vi "STM Read Meta Data (UDP Ref).vi"(6 "Options":T4={"Ignore Timeout Error"=TRUE, "timeout ms (1000)"=1000, "max size (548)"=548}, 8 "error in":errorcluster, 11 "connection ID":refnum<k16>) -> (0 "error out":errorcluster, 1 "Meta data":T1[](array[typedef]), 3 "Connection Info Out":T2, 4 "data info":T3)   [LabVIEW 2010]
doc: "This VI reads the meta data information from a remote computer. Use this VI to retrieve the variable names and types that a remote computer exports.\n\nThis VI parses the data and returns a cluster containing the meta data information.\n\nCopyright 2015, 2016, 2017 National Instruments Corporation\n\nLicensed under the Apache License, Version 2.0 (the \"License\"); you may not use this file except in compliance with the License.\n\n You may obtain a copy of the License at\n\n http://www.apache.org/licenses/LICENSE-2.0\n\nUnless required by applicable law or agreed to in writing, software distributed under the License is distributed on an \"AS IS\" BASIS, WITHOUT WARRANTIES OR CONDITIONS OF ANY KIND, either express or implied.\n\nSee the License for the specific language governing permissions and limitations under the License."
uses:
  stm_UDP Read Options.ctl
  stm_UDP Data Info.ctl
  stm_UDP Connection Info.ctl
  stm_MetaDataElement.ctl
  UDP/Read Meta Data (UDP Clst).vi
  NI STM.lvlib
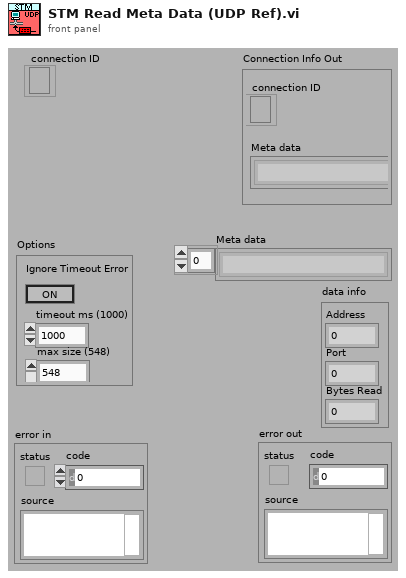
[diagram p1: front panel]
types:
  T1 = typedef "stm_MetaDataElement.ctl" = string
  T2 = typedef "stm_UDP Connection Info.ctl" = cluster{"connection ID":refnum<k16>, "Meta data":T1[]}
  T3 = typedef "stm_UDP Data Info.ctl" = cluster{"Address":u32, "Port":u16, "Bytes Read":i32}
  T4 = typedef "stm_UDP Read Options.ctl" = cluster{"Ignore Timeout Error":bool, "timeout ms (1000)":i32, "max size (548)":i32}
  T5 = typedef "NI STM.lvlib/MetaDataElement.ctl" = string
  T6 = typedef "NI STM.lvlib/UDP Connection Info.ctl" = cluster{"connection ID":refnum<k16>, "meta data":T5[]}
  T7 = typedef "NI STM.lvlib/UDP Data Info.ctl" = cluster{"address":u32, "port":u16, "bytes read":i32}
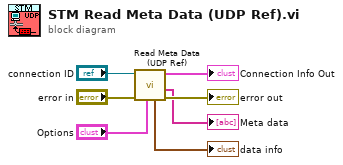
[diagram p0: block diagram]
diagram:
  n1 = call "Read Meta Data (UDP Ref).vi"("options"="Options", "error in"="error in", "connection ID"="connection ID") -> ("error out"=→"error out":errorcluster, "meta data"=→"Meta data":T5[], "connection info out"=→"Connection Info Out":T6, "data info"=→"data info":T7)  [unwired: 5 in]
